vi "Core Actor - CLOSE  - ALL Control References.vi"(8 "error in (no error)":errorcluster, 11 "Child_1_Class in":refnum<class "GUI_Class.lvclass">) -> (0 "error out":errorcluster, 3 "Child_1_Class out":refnum<class "GUI_Class.lvclass">)   [LabVIEW 2023, in "GUI_Actor.lvlib" / "GUI_Class.lvclass"]
uses:
  GUI_Class.lvclass
  GUI_Class.lvclass/GUI_Class.ctl
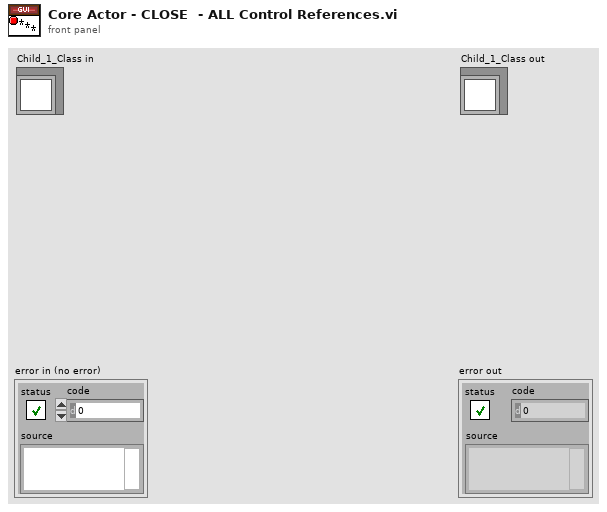
[diagram p1: front panel]
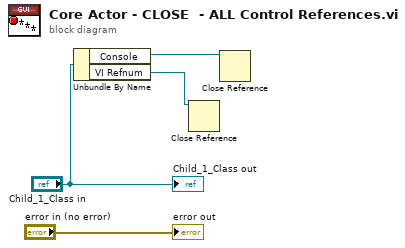
[diagram p0: block diagram]
diagram:
  n1 = Unbundle By Name("Child_1_Class in") -> ("Console"=w3:refnum<vi>, "VI Refnum"=w2:refnum<vi>)
  n2 = Close Reference(reference=w2) -> ()  [unwired: 1 in, 1 out]
  n3 = Close Reference(reference=w3) -> ()  [unwired: 1 in, 1 out]
  "error out" <- "error in (no error)"
  "Child_1_Class out" <- "Child_1_Class in"
